vi "DMA and PIO Write Read.vi"() -> ()   [LabVIEW 2016]
uses:
  <vilib>/Platform/TimedLoop/XDataNode/timing_clust.ctl
  <vilib>/Platform/TimedLoop/XDataNode/nitl_modes.ctl
  <vilib>/Platform/TimedLoop/XDataNode/wakeup.ctl
  Source/GE 5565PIORC/GE 5565PIORC.lvclass/GE 5565PIORC.ctl
  Source/GE 5565PIORC/VIs/Registers/Local Configuration.LAS1RR.Address Range.Get.vi
  Source/GE 5565PIORC/VIs/Registers/Local Configuration.DMACSR0.DMA Enabled.Set.vi
  Source/GE 5565PIORC/VIs/Registers/Local Configuration.INTCSR.Local DMA Interrupt Enable.Set.vi
  Source/GE 5565PIORC/VIs/Registers/Local Configuration.INTCSR.Local Interrupt Input Enable.Set.vi
  Source/GE 5565PIORC/VIs/Registers/Local Configuration.INTCSR.PCI Interrupt Enable.Set.vi
  Source/GE 5565PIORC/VIs/Binary Operations/Align to 8-byte Boundary.vi
  Source/GE 5565PIORC/VIs/Binary Operations/Align to 16-byte Boundary.vi
  Source/GE 5565PIORC/VIs/DMA/DMA.Transfer Size.vi
  Source/GE 5565PIORC/VIs/DMA/DMA.Start Transfer.vi
  Source/GE 5565PIORC/VIs/DMA/DMA.Wait for Done Interrupt Event.vi
  Source/GE 5565PIORC/VIs/Interrupts/Discard PXI Interrupt Events.vi
  Source/GE 5565PIORC/VIs/DMA/DMA.Configure.vi
  Source/GE 5565PIORC/VIs/PIO/SubVIs/PIO.Read Byte Array.vi
  Source/GE 5565PIORC/VIs/Registers/Local Configuration.Get Register Offset.vi
  Source/GE 5565PIORC/VIs/Binary Operations/Set Bits.vi
  Source/GE 5565PIORC/VIs/Binary Operations/Set Bits U32.vi
  Source/GE 5565PIORC/VIs/Registers/Local Configuration.DMACSR0.DMA Start.Set.vi
  Source/GE 5565PIORC/VIs/Interrupts/Wait for PXI Interrupt Events.vi
  Source/GE 5565PIORC/VIs/Registers/Local Configuration.DMACSR0.DMA Clear Interrupt.Set.vi
  <vilib>/Utility/error.llb/Clear Errors.vi
  Source/GE 5565PIORC/VIs/Registers/Local Configuration.PCI Address.Set.vi
  Source/GE 5565PIORC/VIs/Registers/Local Configuration.DMADPR0.First Descriptor Address.Set.vi
  Source/GE 5565PIORC/VIs/DMA/DMA.Scatter-Gather.Link Block Descriptors.vi
  Source/GE 5565PIORC/VIs/DMA/DMA.Scatter-Gather.Commit Blocks.vi
  Source/GE 5565PIORC/VIs/Registers/Local Configuration.Local Address.Set.vi
  Source/GE 5565PIORC/VIs/Registers/Local Configuration.Transfer Size.Set.vi
  Source/GE 5565PIORC/VIs/Registers/Local Configuration.DMADPR0.Transfer Direction.Set.vi
  Source/GE 5565PIORC/VIs/Registers/Local Configuration.DMAMODE0.Scatter-Gather Enable.Set.vi
  Source/GE 5565PIORC/VIs/PIO/SubVIs/PIO.Read U32 Array.vi
  Source/GE 5565PIORC/VIs/PIO/SubVIs/Byte Count to U32 Transfers.vi
  Source/GE 5565PIORC/VIs/PIO/SubVIs/Change Endianness (1D U32).vi
  Source/GE 5565PIORC/VIs/Binary Operations/Get Bits.vi
  Source/GE 5565PIORC/VIs/Binary Operations/Get Bits U32.vi
  Source/GE 5565PIORC/VIs/PIO/SubVIs/Change Endianness (U32).vi
  Source/GE 5565PIORC/GE 5565PIORC.lvclass
  <vilib>/platform/TimedLoop/XDataNode/XDataNode.xnode
  <vilib>/Platform/TimedLoop/XDataNode/XDNodeRunTimeDep.lvlib
panel:
  out "PIO Read":dbl[](array[numeric])
  in  "RFM Offset":u32
  in  "DMA Write":dbl[](array[numeric])=[43264654542.0, 76.0, 738.0]
  in  "VISA resource name":refnum<visa-resource-name>
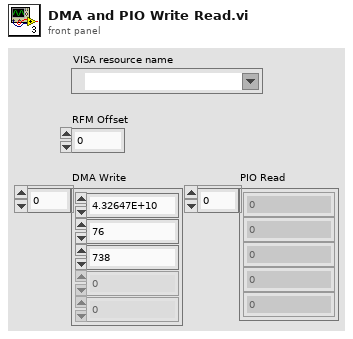
[diagram p1: front panel]
types:
  T1 = typedef "XDNodeRunTimeDep.lvlib/timing_clust.ctl" = cluster{"Expected End [f-1]":u64, "Actual End [f-1]":u64, "Finished Late? [f-1]":bool, "Expected End [i-1]":u64, "Actual End [i-1]":u64, "Finished Late? [i-1]":bool, "Expected Start [i]":u64, "Actual Start [i]":u64, "Expected Start [f]":u64, "Actual Start [f]":u64, "Source Name":string, "Structure Name":string, "Period":i64, "Deadline":i64, "Offset":i64, "Start":i64, "Priority":i32, "Timeout":i32, "Mode":T2, "Wakeup Reason":T3, "Error":errorcluster, "Source Type":string, "Secondary Source Type":string, "Global End Time":u64, "Global Start Time":u64, "Frame Duration":u64, "Iteration Duration":u64, "Assigned CPU":i32, "I/O Scan Engine Mode":u32}
  T2 = typedef "XDNodeRunTimeDep.lvlib/nitl_modes.ctl" = enum32{"No Change", "Process missed periods, maintain original phase", "Discard missed periods, maintain original phase", "Process missed periods, ignore original phase", "Discard missed periods, ignore original phase"}
  T3 = typedef "XDNodeRunTimeDep.lvlib/wakeup.ctl" = enum32{"Normal", "Aborted", "Asynchronous wakeup", "Timing source error", "Timed loop error", "Timeout"}
  T4 = typedef "GE 5565PIORC.lvclass/DMA Block Descriptor.ctl" = cluster{"descriptor ptr (VISA)":u32, "descriptor size":u32, "descriptor ptr (aligned)":u32, "data ptr (lower)":u32, "data ptr (upper)":u32, "data size":u32, "next descriptor ptr":u32}
  T5 = typedef "GE 5565PIORC.lvclass/DMA Transfer Spec.ctl" = cluster{"RFM Address":u32, "Block Descriptors":T4[]}
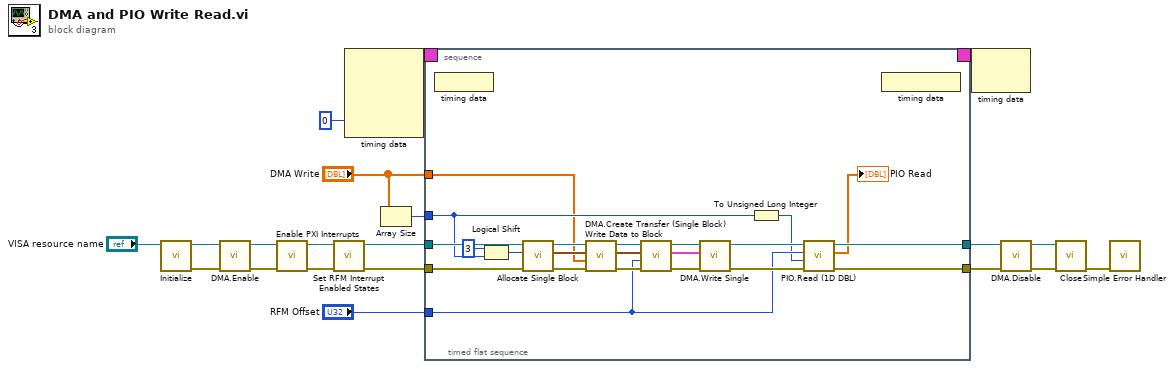
[diagram p0: block diagram]
diagram:
  n1 = call "Initialize.vi"("VISA resource name"="VISA resource name") -> ("error out"=w10:errorcluster, "GE 5565PIORC"=w11:refnum<class "GE 5565PIORC.lvclass">)  [unwired: 9 in]
  n2 = call "DMA.Enable.vi"("error in (no error)"=w10, "GE 5565PIORC in"=w11) -> ("error out"=w14:errorcluster, "GE 5565PIORC out"=w15:refnum<class "GE 5565PIORC.lvclass">)  [unwired: 8 in]
  n3 = call "Enable PXI Interrupts.vi"("error in (no error)"=w14, "GE 5565PIORC in"=w15) -> ("error out"=w12:errorcluster, "GE 5565PIORC out"=w13:refnum<class "GE 5565PIORC.lvclass">)  [unwired: 8 in]
  n4 = call "Set RFM Interrupt Enabled States.vi"("error in (no error)"=w12, "GE 5565PIORC in"=w13) -> ("error out"=w8:errorcluster, "GE 5565PIORC out"=w9:refnum<class "GE 5565PIORC.lvclass">)  [unwired: 8 in]
  n5 = node-c288(0 ("Processor")) -> (w18:T1)  [unwired: 3 in]
  n6 = Array Size(array="DMA Write") -> (size(s)=w5:i32)
  n7 = timed-sequence {
    timing: w18 -> [_]
    timing-out: [_] -> w17
    tunnel: w9 -> [w27]
    tunnel: w8 -> [w26]
    tunnel: w5 -> [w25]
    tunnel: "DMA Write" -> [w24]
    tunnel: "RFM Offset" -> [w23]
    tunnel: [w22] -> w2
    tunnel: [w21] -> w1
    n8 = timed-flat-sequence {
      tunnel: w27 -> [w49]
      tunnel: w26 -> [w48]
      tunnel: w25 -> [w38]
      tunnel: w24 -> [w34]
      tunnel: w23 -> [w30]
      tunnel: [w40] -> w22
      tunnel: [w39] -> w21
      n9 = node-c288() -> ()  [unwired: 1 in]
      n10 = Logical Shift(y=i16 3, x=w38) -> (x << y=w46:i32)
      n11 = call "Allocate Single Block.vi"("error in (no error)"=w48, "size (bytes)"=w46, "GE 5565PIORC in"=w49) -> ("error out"=w36:errorcluster, "Block Descriptor"=w35:T4, "GE 5565PIORC out"=w37:refnum<class "GE 5565PIORC.lvclass">)  [unwired: 6 in]
      n12 = call "Write Data to Block.vi"("error in (no error)"=w36, "Data"=w34, "Block Descriptor"=w35, "GE 5565PIORC"=w37) -> ("error out"=w31:errorcluster, "Block Descriptor out"=w32:T4, "GE 5565PIORC out"=w33:refnum<class "GE 5565PIORC.lvclass">)  [unwired: 5 in]
      n13 = call "DMA.Create Transfer (Single Block).vi"("error in (no error)"=w31, "RFM Offset"=w30, "Block Descriptor"=w32, "GE 5565PIORC in"=w33) -> ("error out"=w43:errorcluster, "DMA Transfer Spec"=w44:T5, "GE 5565PIORC out"=w45:refnum<class "GE 5565PIORC.lvclass">)  [unwired: 4 in, 1 out]
      n14 = call "DMA.Write Single.vi"("error in (no error)"=w43, "DMA Transfer Spec"=w44, "GE 5565PIORC"=w45) -> ("error out"=w41:errorcluster, "GE 5565PIORC out"=w42:refnum<class "GE 5565PIORC.lvclass">)  [unwired: 5 in, 2 out]
      n15 = To Unsigned Long Integer(number=w38) -> (unsigned 32bit integer=w28:u32)
      n16 = call "PIO.Read (1D DBL).vi"("error in (no error)"=w41, "count"=w28, "offset"=w30, "GE 5565PIORC in"=w42) -> ("error out"=w39:errorcluster, "values"=→"PIO Read":dbl[], "GE 5565PIORC out"=w40:refnum<class "GE 5565PIORC.lvclass">)  [unwired: 5 in]
      n17 = node-c288() -> ()  [unwired: 1 out]
    }
  }
  n18 = node-c288(w17) -> ()  [unwired: 1 out]
  n19 = call "DMA.Disable.vi"("error in (no error)"=w1, "GE 5565PIORC in"=w2) -> ("error out"=w6:errorcluster, "GE 5565PIORC out"=w7:refnum<class "GE 5565PIORC.lvclass">)  [unwired: 8 in]
  n20 = call "Close.vi"("error in (no error)"=w6, "GE 5565PIORC in"=w7) -> ("error out"=w19:errorcluster)  [unwired: 8 in, 1 out]
  n21 = call <vilib>:"Simple Error Handler.vi"("error in (no error)"=w19) -> ()  [unwired: 4 in, 5 out]
